vi "Read Action.vi"(8 "error in (no error)":errorcluster, 11 "Action in":refnum<class "Action.lvclass">) -> (0 "error out":errorcluster, 2 "Action":string, 3 "Action out":refnum<class "Action.lvclass">)   [LabVIEW 2013, in "SLMAPI.lvlib" / "Action.lvclass"]
uses:
  Action.lvclass
  Action.lvclass/Action.ctl
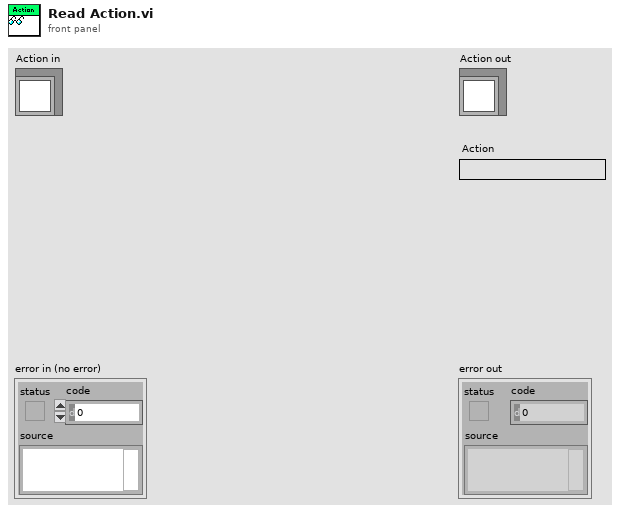
[diagram p1: front panel]
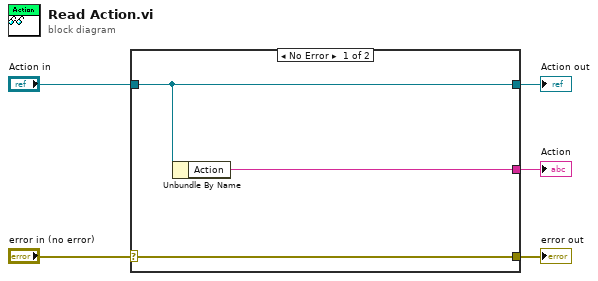
[diagram p0: block diagram]
diagram:
  n1 = case shown="No Error" "error in (no error)" {
    selector: "error in (no error)" -> [w8 w9]
    tunnel: [w8 w9] -> w4
    tunnel: [w7 w10] -> w2
    tunnel: "Action in" -> [w7 w10]
    tunnel: [w6 _] -> w1
    frame No Error {
      n2 = Unbundle By Name(w7) -> ("Action"=w6:string)
    }
    frame Error {
    }
  }
  "error out" <- w4
  "Action out" <- w2
  "Action" <- w1
